vi "RP calculate subset.vi"(5 "Samples per trigger increment":i32=2, 6 "Round off":i32=4096 format="0x%x (%d)", 7 "RAM size":i32=268435456 format="0x%x (%d)", 8 "Trigger start position":i32, 9 "Pre-trigger samples":i32=100000 format="0x%x (%d)", 10 "Bytes per sample":i32, 11 "Post-trigger samples":i32 format="0x%x (%d)") -> (0 "Merged subsets":u64[](array[numeric]) format="0x%x (%d)", 1 "record length":i32 format="0x%x (%d)", 3 "Subsets":i32[][](array[numeric]) format="0x%x (%d)", 4 "pre-trigger trim":i32)   [LabVIEW 2015]
uses:
  Mode.ctl
panel:
  out "post-trigger trim":i32
  out "subset end":i32 format="0x%x (%d)"
  out "subset start":i32 format="0x%x (%d)"
  in  "Mode":T1=enum."Digitizer"
  # "ends"
  # "starts"
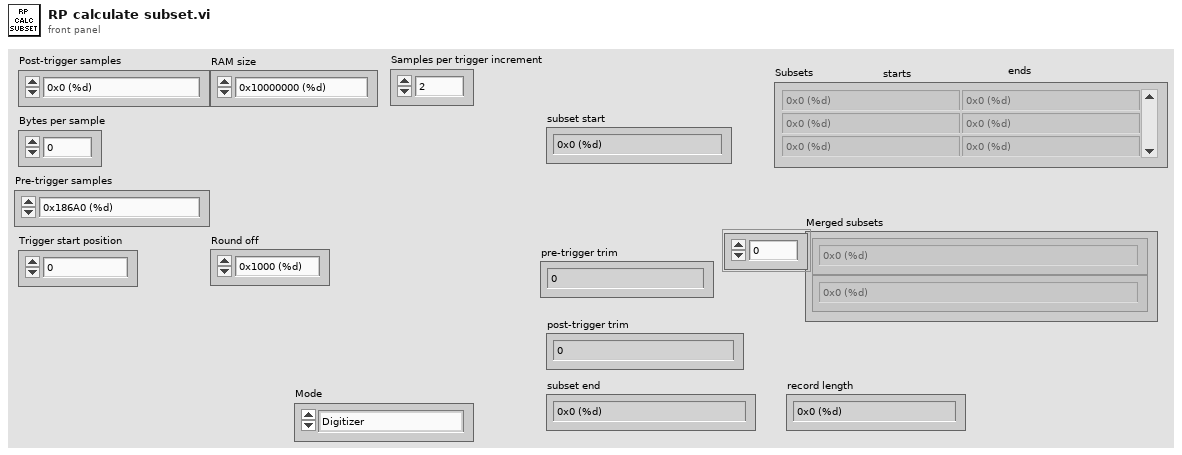
[diagram p1: front panel]
types:
  T1 = typedef "Mode.ctl" = enum16{"Filter", "Lockin test", "Snapshot test", "Digitizer", "Current-Voltage"}
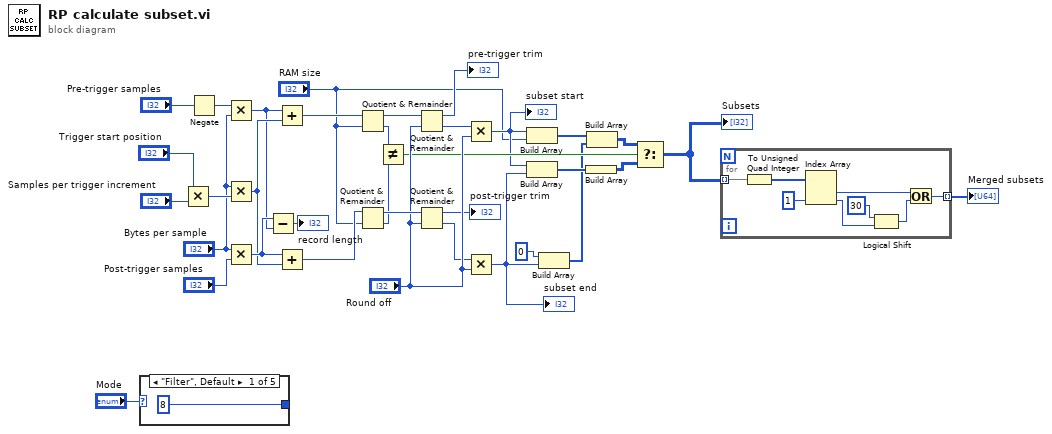
[diagram p0: block diagram]
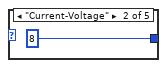
[diagram p2: hidden frame]
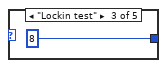
[diagram p3: hidden frame]
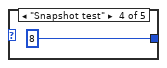
[diagram p4: hidden frame]
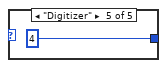
[diagram p5: hidden frame]
diagram:
  n1 = case shown="\"Filter\", Default" "Mode" {
    tunnel: [8 8 8 8 4] -> _
    frame "Filter", Default {
    }
    frame "Current-Voltage" {
    }
    frame "Lockin test" {
    }
    frame "Snapshot test" {
    }
    frame "Digitizer" {
    }
  }
  n2 = Multiply(x="Trigger start position", y="Samples per trigger increment") -> (x*y=w5:i32)
  n3 = Negate(x="Pre-trigger samples") -> (-x=w1:i32)
  n4 = Multiply(x=w1, y="Bytes per sample") -> (x*y=w9:i32)
  n5 = Multiply(x="Bytes per sample", y=w5) -> (x*y=w10:i32)
  n6 = Multiply(x="Bytes per sample", y="Post-trigger samples") -> (x*y=w11:i32)
  n7 = Subtract(x=w11, y=w9) -> (x-y=→"record length":i32)
  n8 = Add(x=w9, y=w10) -> (x+y=w31:i32)
  n9 = Add(x=w11, y=w10) -> (x+y=w33:i32)
  n10 = Quotient & Remainder(x=w31, y="RAM size") -> (x-y*floor(x/y)=w30:i32, floor(x/y)=w24:i32)
  n11 = Quotient & Remainder(x=w33, y="RAM size") -> (x-y*floor(x/y)=w32:i32, floor(x/y)=w23:i32)
  n12 = Not Equal?(x=w24, y=w23) -> (x != y?=w21:bool)
  n13 = Quotient & Remainder(x=w30, y="Round off") -> (x-y*floor(x/y)=→"pre-trigger trim":i32, floor(x/y)=w29:i32)
  n14 = Quotient & Remainder(x=w32, y="Round off") -> (x-y*floor(x/y)=→"post-trigger trim":i32, floor(x/y)=w27:i32)
  n15 = Multiply(x=w29, y="Round off") -> (x*y=w19:i32)
  "subset start" <- w19
  n16 = Multiply(x=w27, y="Round off") -> (x*y=w17:i32)
  "subset end" <- w17
  n17 = Build Array(w19, "RAM size") -> (w15:i32[])
  n18 = Build Array(w19, w17) -> (w22:i32[])
  n19 = Build Array(0 ("element"), w17) -> (w14:i32[])
  n20 = Build Array(w22) -> (w20:i32[][])
  n21 = Build Array(w15, w14) -> (w13:i32[][])
  n22 = Select(t=w13, s=w21, f=w20) -> (s? t:f=w7:i32[][])
  "Subsets" <- w7
  n23 = for {
    tunnel: w7 -> [w48] mode=indexing
    tunnel: [w41] -> w6 mode=indexing
    n24 = To Unsigned Quad Integer(1:w48) -> (0:w47:u64[])
    n25 = Index Array(array=w47, index #2=1 ("index")) -> (element #1=w43:u64, element #2=w45:u64)  [unwired: 1 in]
    n26 = Logical Shift(y=i16 30, x=w45) -> (x << y=w42:u64)
    n27 = Or(x=w43, y=w42) -> (x .or. y?=w41:u64)
  }
  "Merged subsets" <- w6
